vi "Climber_Begin.vi"   [LabVIEW 2012]
uses:
  <vilib>/Rock Robotics/WPI/CAN/Jaguar/SubVIs/WPI_CANJaguar_ControlMode.ctl
  <vilib>/Rock Robotics/WPI/CAN/Jaguar/SubVIs/WPI_CANJaguar_BrakeCoastMode.ctl
  <vilib>/Rock Robotics/WPI/MotorControl/WPI_MotorControlOpenCANJaguar.vi
types:
  T1 = typedef "WPI_CANJaguar_BrakeCoastMode.ctl" = enum8{"Jumper", "Brake", "Coast"}
  T2 = typedef "WPI_CANJaguar_ControlMode.ctl" = enum8{"Percent VBus", "Current", "Speed", "Position", "Voltage"}
  T3 = typedef "WPI_MotorControlDeviceRef.ctl" = cluster{"DeviceStatus":errorcluster, "Type":enum16{"PWM", "CAN"}, "PWM":cluster{"Digital Module":T4, "PWM Channel":T5, "DeadBand":T6}, "CAN":cluster{"Device Number":u8, "Control Mode":T2, "Semaphore":T7, "Max Vout":dbl}, "Invert":bool, "TransformRef":T8, "InvTransformRef":T8}
  T4 = typedef "FPGA_TypedefDigitalModule.ctl" = enum16{"Digital Module 1", "Digital Module 2"}
  T5 = typedef "FPGA_DIOPWMChannel.ctl" = enum8{"PWM 1", "PWM 2", "PWM 3", "PWM 4", "PWM 5", "PWM 6", "PWM 7", "PWM 8", "PWM 9", "PWM 10", "Invalid"}
  T6 = typedef "WPI_PWMDeadband.ctl" = cluster{"Name":string, "maxPositivePwm":i32, "minPositivePwm":i32, "centerPwm":i32, "maxNegativePwm":i32, "minNegativePwm":i32, "angularRange":u16}
  T7 = typedef "Semaphore RefNum" = refnum<k1>
  T8 = typedef "WPI_PWMTransform_ConPane.ctl" = refnum<vi>
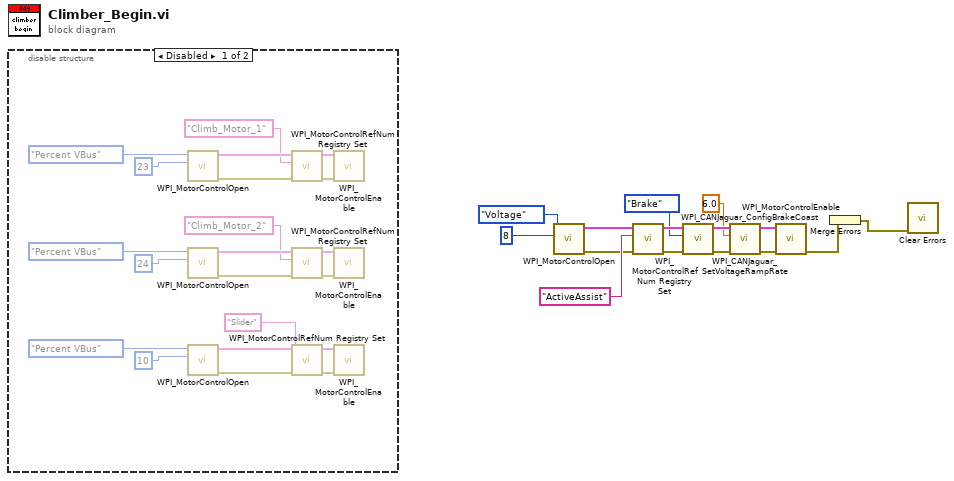
[diagram p0: block diagram]
diagram:
  n1 = disable-structure shown="Disabled" {
    frame Disabled {
      n2 = call-poly <vilib>:"WPI_MotorControlOpen.vi"("Device Number"=u8 23, "Control Mode"=WPI_CANJaguar_ControlMode."Percent VBus") -> ("error out"=w36:errorcluster, "MotorControlDeviceRef"=w35:T3)  [unwired: 8 in]
      n3 = call-poly <vilib>:"WPI_MotorControlOpen.vi"("Device Number"=u8 24, "Control Mode"=WPI_CANJaguar_ControlMode."Percent VBus") -> ("error out"=w34:errorcluster, "MotorControlDeviceRef"=w33:T3)  [unwired: 8 in]
      n4 = call-poly <vilib>:"WPI_MotorControlOpen.vi"("Device Number"=u8 10, "Control Mode"=WPI_CANJaguar_ControlMode."Percent VBus") -> ("error out"=w18:errorcluster, "MotorControlDeviceRef"=w17:T3)  [unwired: 8 in]
      n5 = call <vilib>:"WPI_MotorControlRefNum Registry Set.vi"("error in (no error)"=w36, "refnum name"="Climb_Motor_1", "MotorControlDevRef"=w35) -> ("error out"=w30:errorcluster, "MotorControlDevRef"=w29:T3)  [unwired: 7 in]
      n6 = call <vilib>:"WPI_MotorControlRefNum Registry Set.vi"("error in (no error)"=w34, "refnum name"="Climb_Motor_2", "MotorControlDevRef"=w33) -> ("error out"=w27:errorcluster, "MotorControlDevRef"=w28:T3)  [unwired: 7 in]
      n7 = call <vilib>:"WPI_MotorControlRefNum Registry Set.vi"("error in (no error)"=w18, "refnum name"="Slider", "MotorControlDevRef"=w17) -> ("error out"=w19:errorcluster, "MotorControlDevRef"=w20:T3)  [unwired: 7 in]
      n8 = call <vilib>:"WPI_MotorControlEnable.vi"("error in (no error)"=w30, "CAN Jaguar Ref"=w29) -> ()  [unwired: 8 in, 2 out]
      n9 = call <vilib>:"WPI_MotorControlEnable.vi"("error in (no error)"=w27, "CAN Jaguar Ref"=w28) -> ()  [unwired: 8 in, 2 out]
      n10 = call <vilib>:"WPI_MotorControlEnable.vi"("error in (no error)"=w19, "CAN Jaguar Ref"=w20) -> ()  [unwired: 8 in, 2 out]
    }
    frame Enabled {
    }
  }
  n11 = call-poly <vilib>:"WPI_MotorControlOpen.vi"("Device Number"=u8 8, "Control Mode"=WPI_CANJaguar_ControlMode."Voltage") -> ("error out"=w12:errorcluster, "MotorControlDeviceRef"=w15:T3)  [unwired: 8 in]
  n12 = call <vilib>:"WPI_MotorControlRefNum Registry Set.vi"("error in (no error)"=w12, "refnum name"="ActiveAssist", "MotorControlDevRef"=w15) -> ("error out"=w9:errorcluster, "MotorControlDevRef"=w13:T3)  [unwired: 7 in]
  n13 = call <vilib>:"WPI_CANJaguar_ConfigBrakeCoast.vi"("error in (no error)"=w9, "Brake / Coast Mode"=WPI_CANJaguar_BrakeCoastMode."Brake", "CAN Jaguar Ref"=w13) -> ("error out"=w2:errorcluster, "CAN Jaguar Ref Out"=w3:T3)  [unwired: 7 in]
  n14 = call <vilib>:"WPI_CANJaguar_SetVoltageRampRate.vi"("error in (no error)"=w2, "VoltageRampRate (V/s)"=6.0, "CAN Jaguar Ref"=w3) -> ("error out"=w5:errorcluster, "CAN Jaguar Ref Out"=w4:T3)  [unwired: 7 in]
  n15 = call <vilib>:"WPI_MotorControlEnable.vi"("error in (no error)"=w5, "CAN Jaguar Ref"=w4) -> ("error out"=w7:errorcluster)  [unwired: 8 in, 1 out]
  n16 = Merge Errors(w7) -> (w6:errorcluster)
  n17 = call <vilib>:"Clear Errors.vi"("error in (no error)"=w6) -> ()  [unwired: 6 in, 1 out]
